vi "Generate Motion Profile From Acceleration.vi"(6 "Initial Velocity (in/s)":dbl, 7 "Time Between Points (ms)":dbl, 8 "Error In":errorcluster, 9 "Movement Duration (s)":dbl, 10 "Acceleration (in/s2)":dbl, 11 "Initial Position (in)":dbl) -> (0 "Error Out":errorcluster, 2 "Duration (s)":dbl, 3 "Motion Profile Portion":T1[](array[typedef]))   [LabVIEW 2019, in "Motion Profile Generator.lvclass"]
uses:
  Motion Profile Generator.lvclass
  Type Defs/Motion Profile Point.ctl
  <vilib>/ErrorRing/Error Ring.xnode
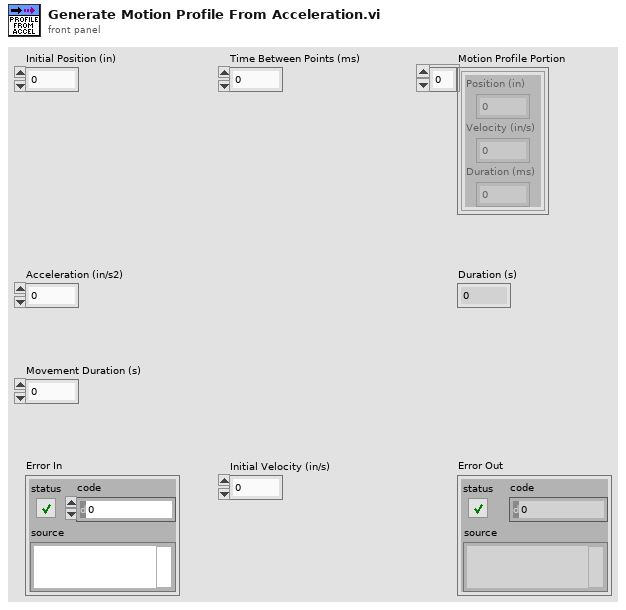
[diagram p1: front panel]
types:
  T1 = typedef "Motion Profile Generator.lvclass/Motion Profile Point.ctl" = cluster{"Position (in)":dbl, "Velocity (in/s)":dbl, "Duration (ms)":dbl}
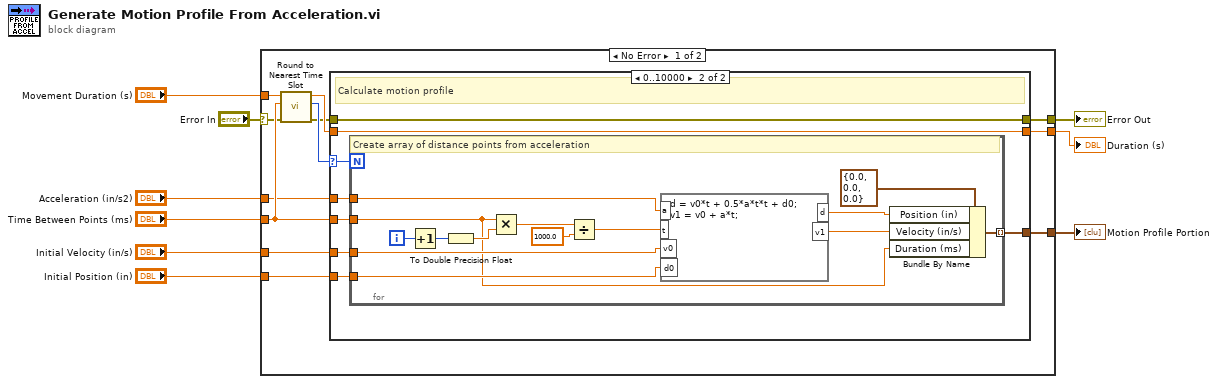
[diagram p0: block diagram]
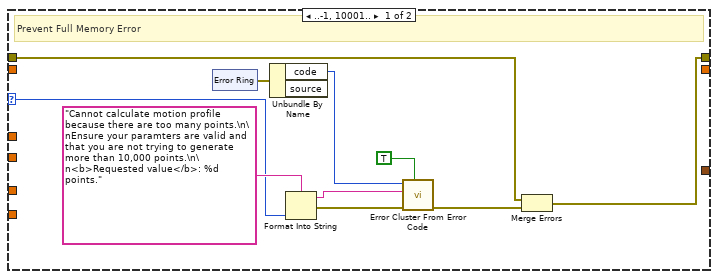
[diagram p2: hidden frame]
diagram:
  n1 = case shown="No Error" "Error In" {
    selector: "Error In" -> [w11 w58]
    tunnel: [w21 _] -> w9
    tunnel: "Initial Position (in)" -> [w20 _]
    tunnel: "Movement Duration (s)" -> [w19 _]
    tunnel: "Initial Velocity (in/s)" -> [w18 _]
    tunnel: "Time Between Points (ms)" -> [w17 _]
    tunnel: "Acceleration (in/s2)" -> [w16 _]
    tunnel: [w14 w58] -> w3
    tunnel: [w13 _] -> w1
    frame No Error {
      n2 = call "Round to Nearest Time Slot.vi"("Error In"=w11, "Time Slot Size (ms)"=w17, "Duration (s)"=w19) -> ("Error Out"=w10:errorcluster, "Slots Count"=w15:i32, "Nearest Time Slot (s)"=w12:dbl)  [unwired: 6 in]
      n3 = case shown="0..10000" w15 {
        selector: w15 -> [w22 w38]
        tunnel: [_ w43] -> w21
        tunnel: w20 -> [_ w42]
        tunnel: w18 -> [_ w41]
        tunnel: w17 -> [_ w40]
        tunnel: w16 -> [_ w39]
        tunnel: [w30 w37] -> w14
        tunnel: w10 -> [w31 w37]
        tunnel: [_ w36] -> w13
        tunnel: w12 -> [_ w36]
        frame ..-1, 10001.. {
          # "Prevent Full Memory Error"
          n4 = xnode "Error Ring"() -> ("error out"=w28:errorcluster)
          n5 = Unbundle By Name(w28) -> ("code"=w27:i32)  [unwired: 1 out]
          n6 = Format Into String(format string="Cannot calculate motion profile because there are too many points.\n\nEnsure your paramters are valid and that you are not trying to generate more than 10,000 points.\n\n<b>Requested value</b>: %d points." ("error message (\"\")"), w22) -> (resulting string=w24:string, error out=w25:errorcluster)  [unwired: 2 in]
          n7 = call <vilib>:"Error Cluster From Error Code.vi"("show call chain? (False)"=TRUE, "error in (no error)"=w25, "error message (\"\")"=w24, "error code (0)"=w27) -> ("error out"=w29:errorcluster)  [unwired: 5 in]
          n8 = Merge Errors(w31, w29) -> (w30:errorcluster)
        }
        frame 0..10000 {
          # "Calculate motion profile"
          n9 = for {
            N: w38 -> [_]
            tunnel: w39 -> [w57]
            tunnel: w40 -> [w45]
            tunnel: w41 -> [w52]
            tunnel: w42 -> [w49]
            tunnel: [w44] -> w43 mode=indexing
            i -> [w56]
            # "Create array of distance points from acceleration"
            n10 = Increment(x=w56) -> (x+1=w55:i32)
            n11 = To Double Precision Float(number=w55) -> (double precision float=w51:dbl)
            n12 = Multiply(x=w45, y=w51) -> (x*y=w54:dbl)
            n13 = Divide(x=w54, y=1000.0) -> (x/y=w50:dbl)
            n14 = formula code="d = v0*t + 0.5*a*t*t + d0;\nv1 = v0 + a*t;"("a"=w57, "v0"=w52, "t"=w50, "d0"=w49) -> ("d"=w47:dbl, "v1"=w46:dbl)
            n15 = Bundle By Name(cluster=T1 {"Position (in)"=0.0, "Velocity (in/s)"=0.0, "Duration (ms)"=0.0} ("Motion Profile Point"), "Position (in)"=w47, "Velocity (in/s)"=w46, "Duration (ms)"=w45) -> (w44:T1)
          }
        }
      }
    }
    frame Error {
    }
  }
  "Motion Profile Portion" <- w9
  "Duration (s)" <- w1
  "Error Out" <- w3
